vi "Get Paths.vi"(8 "error in":errorcluster, 10 "Naming Data":refnum<class "Naming Data.lvclass">, 11 "Namer with Folder in":refnum<class "Namer with Folder.lvclass">) -> (0 "error out":errorcluster, 1 "Received Path":path, 2 "Approved Path":path, 3 "Namer with Folder out":refnum<class "Namer with Folder.lvclass">)   [LabVIEW 2020, in "Approval Tests.lvlib" / "Namer with Folder.lvclass"]
uses:
  Namer with Folder.lvclass
  Naming Data/Naming Data.lvclass
  Namer with Folder.lvclass/Namer with Folder.ctl
  Namer Decorator/Namer Decorator.lvclass
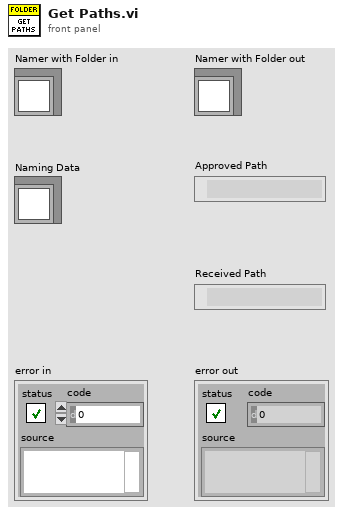
[diagram p1: front panel]
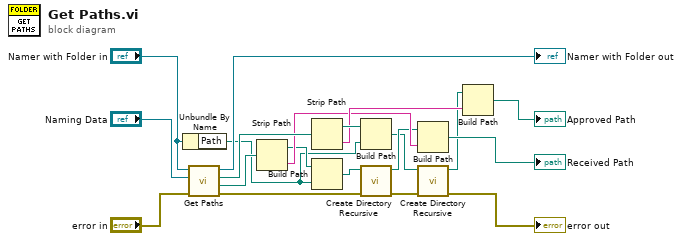
[diagram p0: block diagram]
diagram:
  n1 = Unbundle By Name("Namer with Folder in") -> ("Path"=w5:path)
  n2 = call-parent "Get Paths.vi"("error in"="error in", "Naming Data"="Naming Data", "Namer Decorator in"="Namer with Folder in") -> ("error out"=w19:errorcluster, "Received Path"=w14:path, "Approved Path"=w12:path, "Namer Decorator out"=→"Namer with Folder out":refnum<class "Namer with Folder.lvclass">)  [unwired: 5 in]
  n3 = Strip Path(path=w14) -> (stripped path=w6:path, name=w7:string)
  n4 = Strip Path(path=w12) -> (stripped path=w9:path, name=w8:string)
  n5 = Build Path(base path=w6, name or relative path=w5) -> (appended path=w3:path)
  n6 = Build Path(base path=w9, name or relative path=w5) -> (appended path=w2:path)
  n7 = call <vilib>:"Create Directory Recursive.vi"("error in (no error)"=w19, "directory"=w3) -> ("error out"=w18:errorcluster, "directory copy"=w4:path)  [unwired: 3 in, 1 out]
  n8 = Build Path(base path=w4, name or relative path=w7) -> (appended path=→"Received Path":path)
  n9 = call <vilib>:"Create Directory Recursive.vi"("error in (no error)"=w18, "directory"=w2) -> ("error out"=→"error out":errorcluster, "directory copy"=w1:path)  [unwired: 3 in, 1 out]
  n10 = Build Path(base path=w1, name or relative path=w8) -> (appended path=→"Approved Path":path)
